vi "BG correction.vi"(7 "Change?":bool, 8 "error in (no error)":errorcluster, 9 "def pixel upper":i32, 10 "def pixel lower":i32, 11 "Control-Client in":refnum<class "Control-Client.lvclass">) -> (0 "error out":errorcluster, 3 "Control-Client out":refnum<class "Control-Client.lvclass">)   [LabVIEW 2020, in "Control-Client.lvclass"]
uses:
  Control-Client.lvclass
  Control-Client.lvclass/Control-Client.ctl
  Experiments/Experiment.lvclass
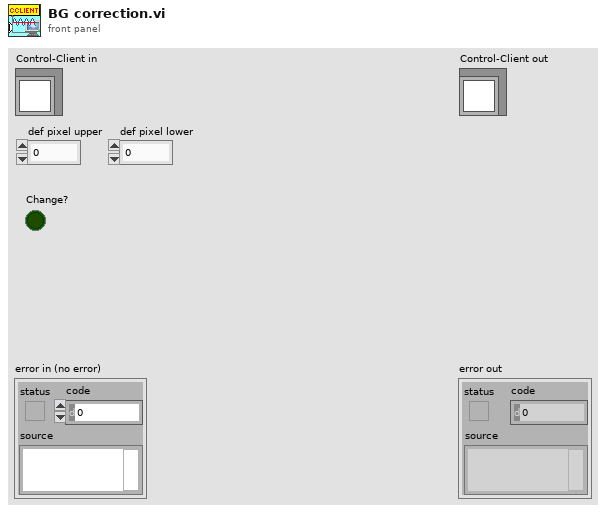
[diagram p1: front panel]
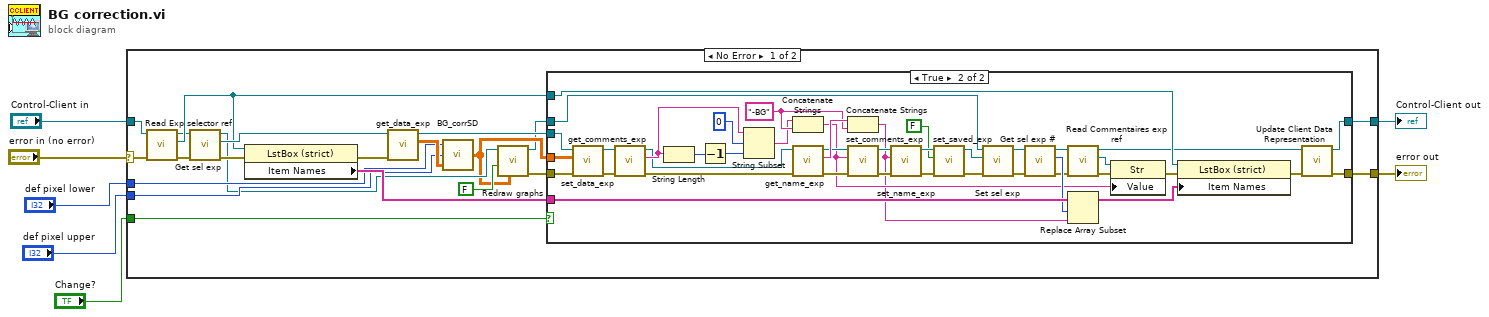
[diagram p0: block diagram]
diagram:
  n1 = case shown="No Error" "error in (no error)" {
    selector: "error in (no error)" -> [w27 w73]
    tunnel: [w19 w73] -> w6
    tunnel: [w18 w72] -> w4
    tunnel: "Control-Client in" -> [w26 w72]
    tunnel: "def pixel lower" -> [w21 _]
    tunnel: "def pixel upper" -> [w20 _]
    tunnel: "Change?" -> [w8 _]
    frame No Error {
      n2 = call "Read Exp selector ref.vi"("error in (no error)"=w27, "Control-Client in"=w26) -> ("error out"=w13:errorcluster, "Exp selector ref"=w24:refnum<vi>, "Control-Client out"=w14:refnum<class "Control-Client.lvclass">)  [unwired: 7 in]
      n3 = call "Get sel exp.vi"("error in (no error)"=w13, "Control-Client in"=w14) -> ("error out"=w23:errorcluster, "Sel experiment"=w28:refnum<class "Experiment.lvclass">, "Control-Client out"=w17:refnum<class "Control-Client.lvclass">)  [unwired: 7 in]
      n4 = property on="Property Node" class="LstBox (strict)"(reference=w24, error in=w23) -> (error out=w16:errorcluster, "Item Names"=w25:string[])  [unwired: 1 out]
      n5 = call "get_data_exp.vi"("error in (no error)"=w16, "Experiment.lvclass in"=w28) -> ("Data"=w22:sgl[][], "Experiment.lvclass out"=w10:refnum<class "Experiment.lvclass">)  [unwired: 7 in, 1 out]
      n6 = call "BG_corrSD.vi"("Data"=w22, "upper pixel"=w20, "lower pixel"=w21) -> ("Data corrected"=w12:dbl[][])
      n7 = call "Redraw graphs.vi"("Data"=w12, "Selected exp"=FALSE, "Control-Client in"=w17) -> ("error out"=w11:errorcluster, "Control-Client out"=w9:refnum<class "Control-Client.lvclass">)  [unwired: 7 in]
      n8 = case shown="True" w8 {
        tunnel: w25 -> [_ w71]
        tunnel: w24 -> [_ w70]
        tunnel: [w29 w69] -> w19
        tunnel: [w30 w68] -> w18
        tunnel: w12 -> [_ w38]
        tunnel: w11 -> [w29 w33]
        tunnel: w10 -> [_ w32]
        tunnel: w9 -> [w30 w31]
        frame False {
        }
        frame True {
          w60 = "-BG" ("string")
          n9 = call "set_data_exp.vi"("error in (no error)"=w33, "Data"=w38, "Experiment.lvclass in"=w32) -> ("error out"=w44:errorcluster, "Experiment.lvclass out"=w45:refnum<class "Experiment.lvclass">)  [unwired: 7 in]
          n10 = call "get_comments_exp.vi"("error in (no error)"=w44, "Experiment.lvclass in"=w45) -> ("error out"=w66:errorcluster, "Comments"=w58:string, "Experiment.lvclass out"=w47:refnum<class "Experiment.lvclass">)  [unwired: 7 in]
          n11 = String Length(string=w58) -> (length=w56:i32)
          n12 = Decrement(x=w56) -> (x-1=w55:i32)
          n13 = String Subset(string=w58, offset (0)=0, length (rest)=w55) -> (substring=w54:string)
          n14 = Concatenate Strings(w54, w60) -> (w37:string)
          n15 = call "get_name_exp.vi"("error in (no error)"=w66, "Experiment.lvclass in"=w47) -> ("error out"=w67:errorcluster, "Exp name"=w65:string, "Experiment.lvclass out"=w46:refnum<class "Experiment.lvclass">)  [unwired: 7 in]
          n16 = Concatenate Strings(w65, w60) -> (w36:string)
          n17 = call "set_comments_exp.vi"("error in (no error)"=w67, "Comments"=w37, "Experiment.lvclass in"=w46) -> ("error out"=w63:errorcluster, "Experiment.lvclass out"=w64:refnum<class "Experiment.lvclass">)  [unwired: 7 in]
          n18 = call "set_name_exp.vi"("error in (no error)"=w63, "Exp name"=w36, "Experiment.lvclass in"=w64) -> ("error out"=w61:errorcluster, "Experiment.lvclass out"=w62:refnum<class "Experiment.lvclass">)  [unwired: 7 in]
          n19 = call "set_saved_exp.vi"("error in (no error)"=w61, "Saved"=FALSE, "Experiment.lvclass in"=w62) -> ("error out"=w34:errorcluster, "Experiment.lvclass out"=w35:refnum<class "Experiment.lvclass">)  [unwired: 7 in]
          n20 = call "Set sel exp.vi"("error in (no error)"=w34, "Experiment"=w35, "Control-Client in"=w31) -> ("error out"=w41:errorcluster, "Control-Client out"=w48:refnum<class "Control-Client.lvclass">)  [unwired: 7 in]
          n21 = call "Get sel exp #.vi"("error in (no error)"=w41, "Control-Client in"=w48) -> ("error out"=w40:errorcluster, "Exp sel #"=w52:i32, "Control-Client out"=w43:refnum<class "Control-Client.lvclass">)  [unwired: 7 in]
          n22 = call "Read Commentaires exp ref.vi"("error in (no error)"=w40, "Control-Client in"=w43) -> ("error out"=w50:errorcluster, "Commentaires exp ref"=w51:refnum<vi>, "Control-Client out"=w42:refnum<class "Control-Client.lvclass">)  [unwired: 7 in]
          n23 = Replace Array Subset(array=w71, new element=w36, index=w52) -> (w53:string[])
          n24 = property on="Property Node" class="Str"(reference=w51, error in=w50, "Value"=w37) -> (error out=w49:errorcluster)  [unwired: 1 out]
          n25 = property on="Property Node" class="LstBox (strict)"(reference=w70, error in=w49, "Item Names"=w53) -> (error out=w39:errorcluster)  [unwired: 1 out]
          n26 = call "Update Client Data Representation.vi"("error in (no error)"=w39, "Control-Client in"=w42) -> ("error out"=w69:errorcluster, "Control-Client out"=w68:refnum<class "Control-Client.lvclass">)  [unwired: 8 in]
        }
      }
    }
    frame Error {
    }
  }
  "error out" <- w6
  "Control-Client out" <- w4
